vi "Main.vi"(8 "error in":errorcluster, 11 "TCP Client in":refnum<class "TCP Client.lvclass">) -> (0 "error out":errorcluster, 3 "TCP Client out":refnum<class "TCP Client.lvclass">)   [LabVIEW 2017, in "TCP Client.lvlib" / "TCP Client.lvclass"]
doc: "The <b>Queued Message Handler</b> of the Worker that owns this VI."
uses:
  TCP Client.lvclass
  C:/Program Files (x86)/National Instruments/LabVIEW 2017/vi.lib/addons/_Workers/Library/Classes/Worker/Worker.lvclass
  Initialization Data.ctl
  Response Cases.ctl
  <vilib>/addons/_Workers/Library/Case Label.ctl
  TCP Client.lvclass/TCP Client.ctl
  rql_New Connection.ctl
  <vilib>/addons/_Workers/Library/Classes/Message/Priority.ctl
  rsp_Connection Notify.ctl
  rql_Create Read Worker.ctl
  TCP Read/Initialization Data.ctl
  TCP Read/Response Cases.ctl
  <vilib>/addons/_Workers/Library/Classes/Message Queue/Message Queue.lvclass
  rwr_Connect to Server.ctl
  rqp_Send String to Server.ctl
  <vilib>/Utility/error.llb/Error Cluster From Error Code.vi
  <vilib>/ErrorRing/Error Ring.xnode
  <vilib>/addons/_Workers/Library/Classes/Worker/Worker.lvclass
  <vilib>/addons/_Workers/Library/Workers.lvlib
  <vilib>/addons/_Workers/Library/Classes/Message/Message.lvclass
  TCP Read/TCP Read.lvclass
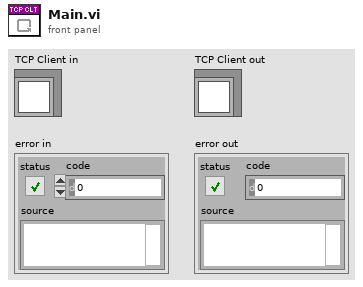
[diagram p1: front panel]
types:
  T1 = typedef "TCP Client.lvlib/TCP Client.lvclass/Initialization Data.ctl" = cluster{"Response Cases":T2}
  T2 = typedef "TCP Client.lvlib/TCP Client.lvclass/Response Cases.ctl" = cluster{"Connection Notify":T3, "Incoming Data":T3}
  T3 = typedef "Workers.lvlib/Case Label.ctl" = string
  T4 = typedef "TCP Client.lvlib/TCP Client.lvclass/rsp_Connection Notify.ctl" = cluster{"Server Name":string, "IP Address":string, "Connected?":bool}
  T5 = typedef "Workers.lvlib/Message.lvclass/Priority.ctl" = enum16{"Low", "Normal", "High"}
  T6 = typedef "TCP Client.lvlib/TCP Client.lvclass/rql_New Connection.ctl" = cluster{"Connection ID":refnum<k5>, "Server Name":string, "IP Address":string}
  T7 = typedef "TCP Client.lvlib/TCP Read.lvclass/Initialization Data.ctl" = cluster{"Response Cases":T8, "Connection ID":refnum<k5>, "Forwarding Queue":refnum<class "Message Queue.lvclass">, "Forwarding Case":T3, "Server Name":string}
  T8 = typedef "TCP Client.lvlib/TCP Read.lvclass/Response Cases.ctl" = cluster{"Connection Lost":T3}
  T9 = typedef "TCP Client.lvlib/TCP Client.lvclass/rql_Create Read Worker.ctl" = cluster{"String":string}
  T10 = typedef "TCP Client.lvlib/TCP Client.lvclass/rwr_Connect to Server.ctl" = cluster{"Client Name":string, "Server IP Address":string, "Server Port":u16}
  T11 = typedef "TCP Client.lvlib/TCP Client.lvclass/rqp_Send String to Server.ctl" = cluster{"String to Send":string}
  T12 = typedef "TCP Client.lvlib/TCP Read.lvclass/rsp_Connection Lost.ctl" = cluster{"Connection ID":refnum<k5>, "TCP Read Queue":refnum<class "Message Queue.lvclass">}
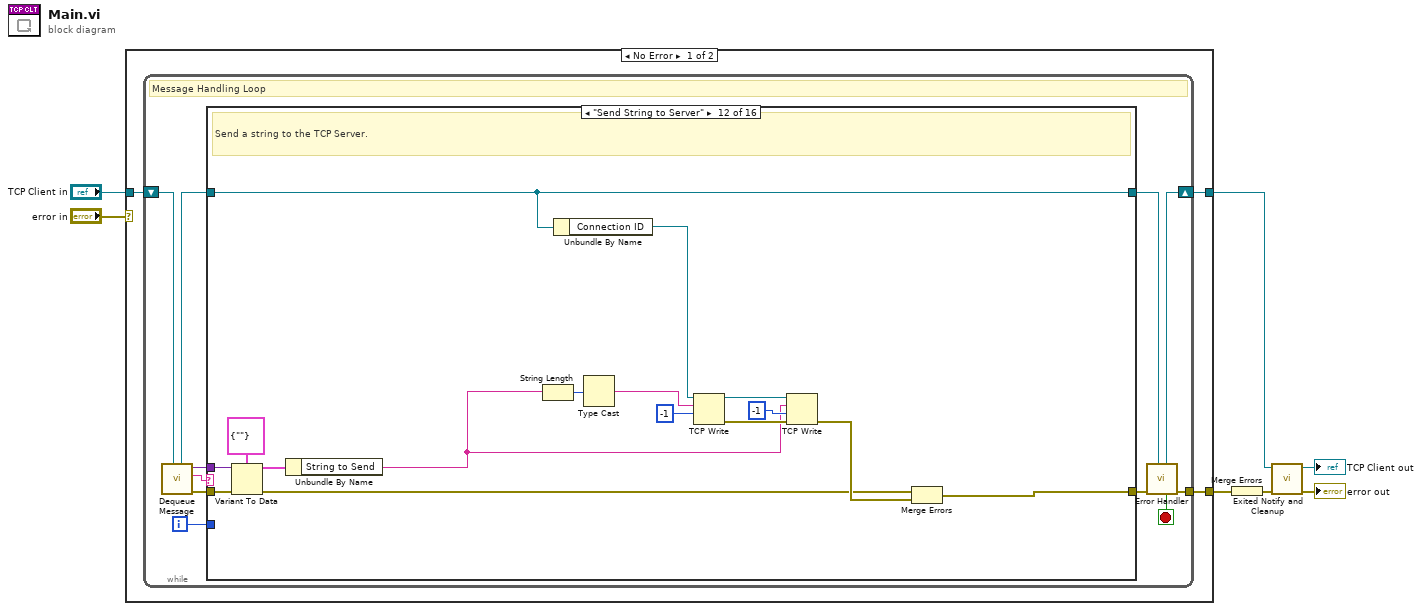
[diagram p0: block diagram]
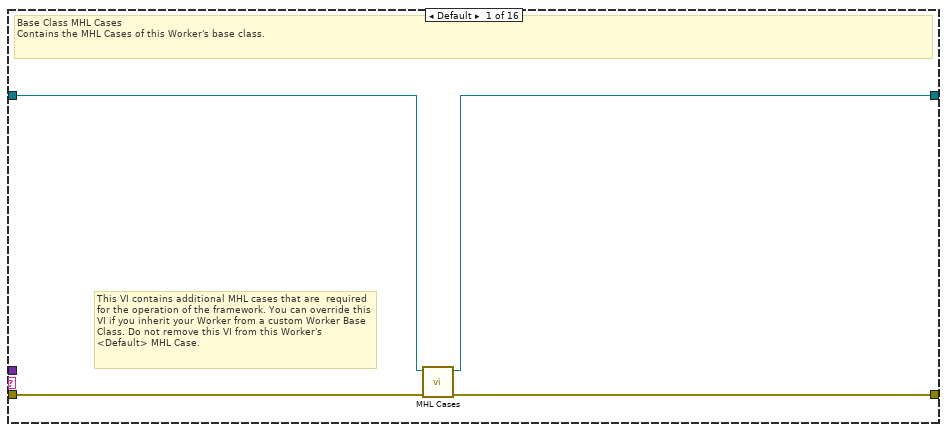
[diagram p2: hidden frame]
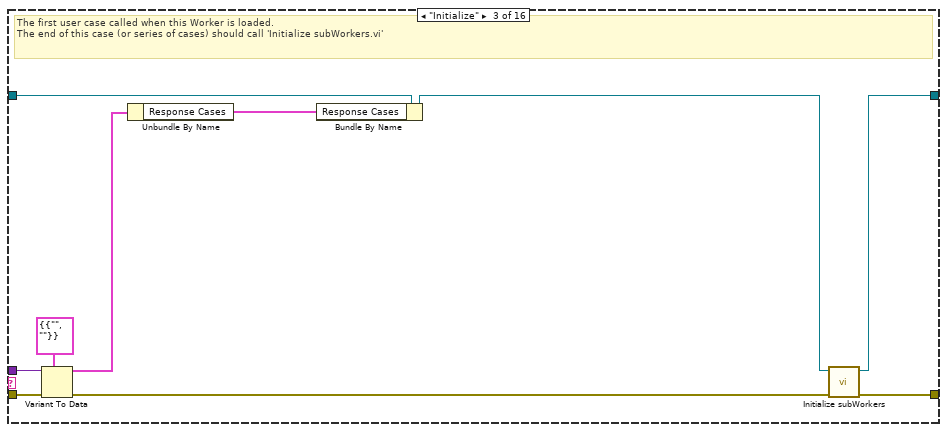
[diagram p4: hidden frame]
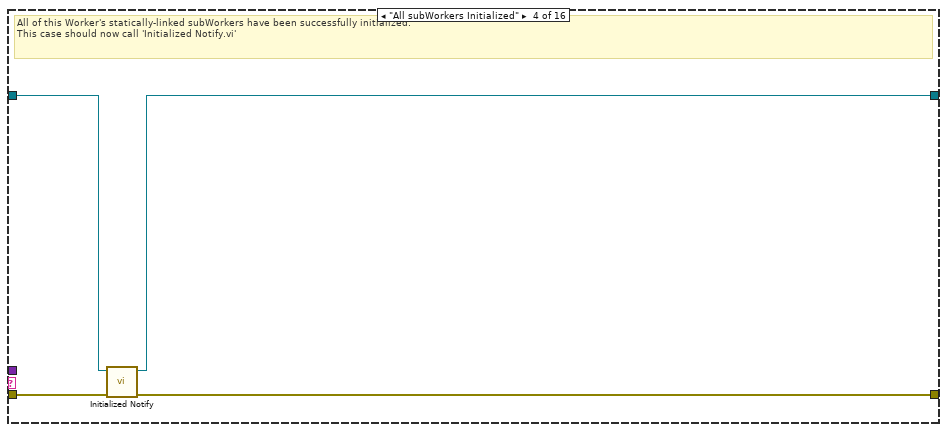
[diagram p5: hidden frame]
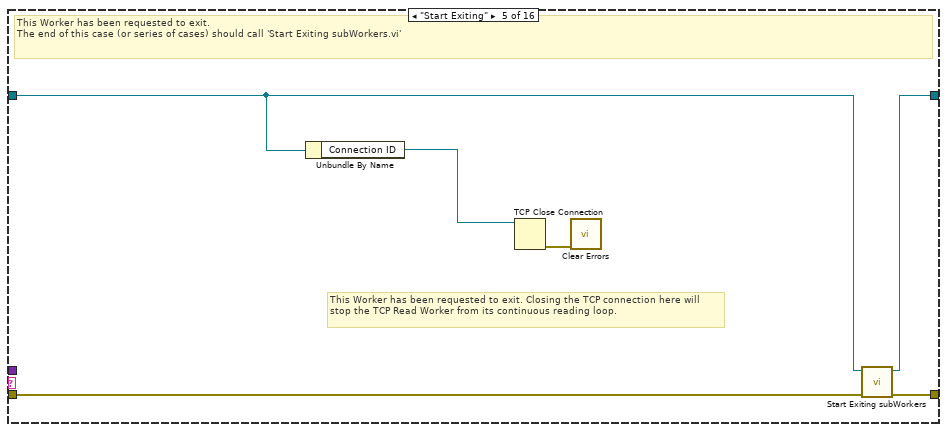
[diagram p6: hidden frame]
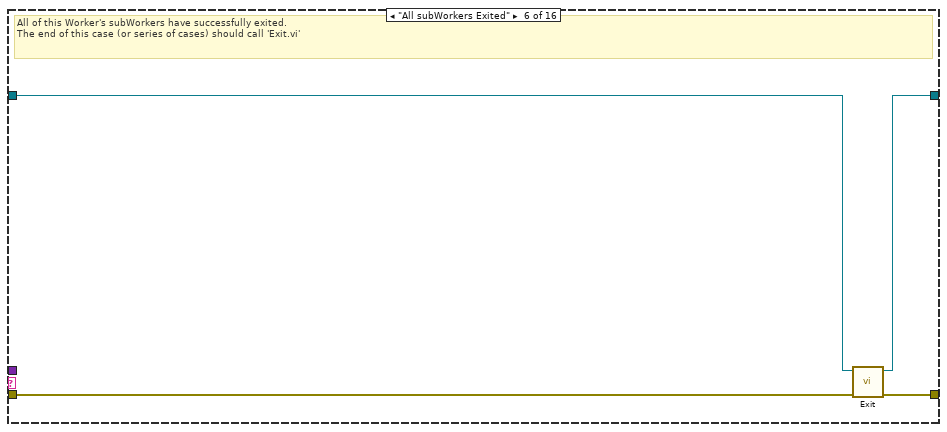
[diagram p7: hidden frame]
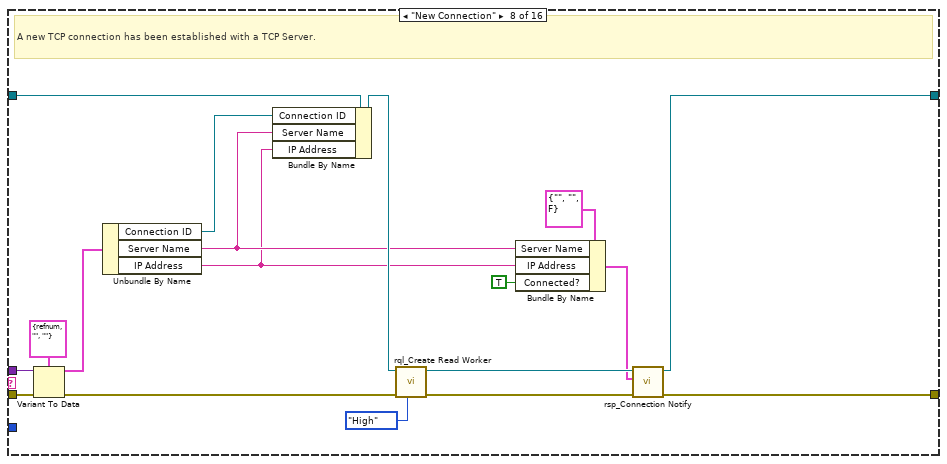
[diagram p9: hidden frame]
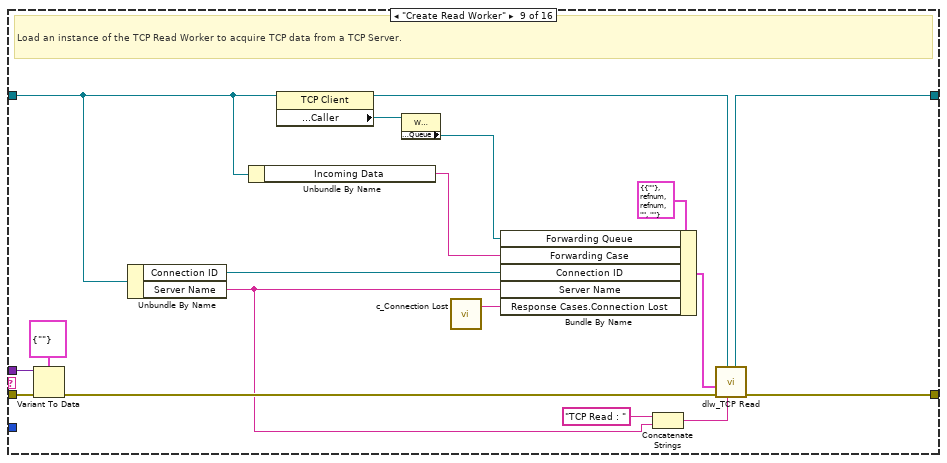
[diagram p10: hidden frame]
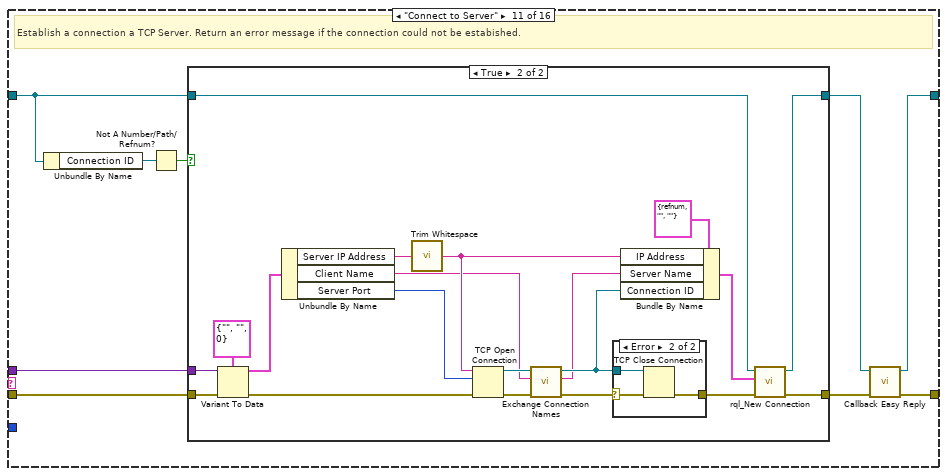
[diagram p12: hidden frame]
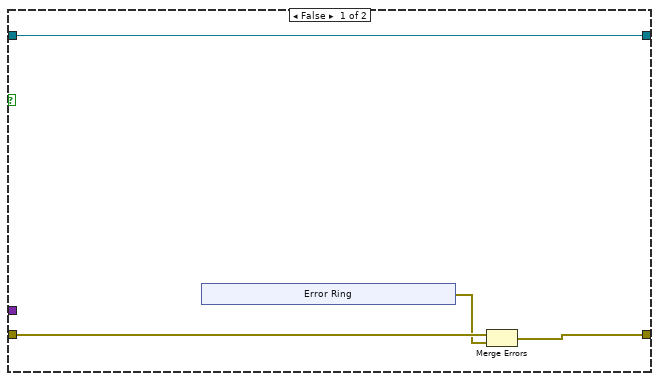
[diagram p13: hidden frame]
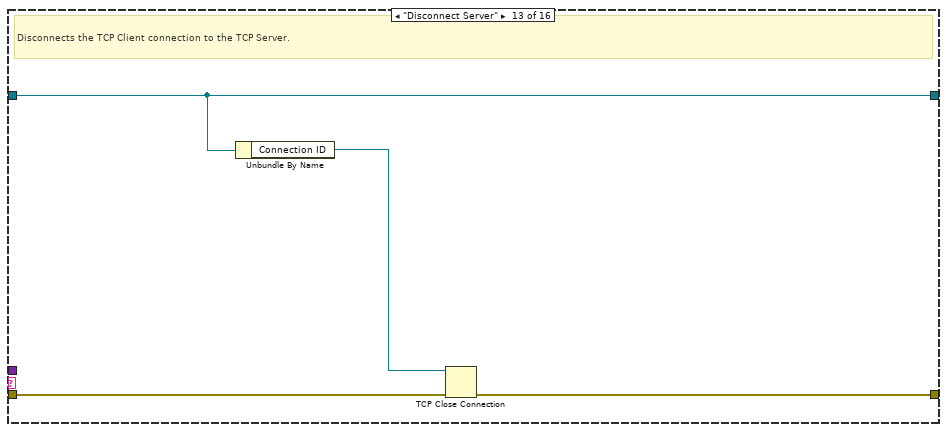
[diagram p15: hidden frame]
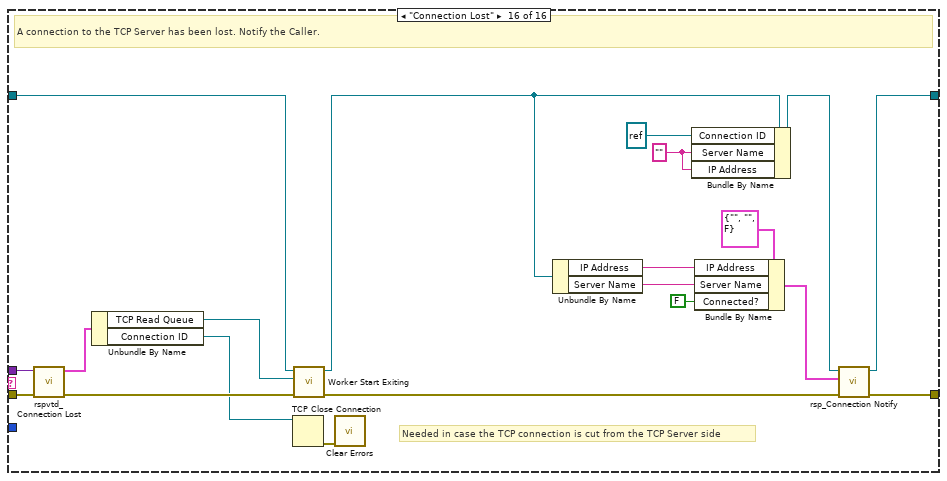
[diagram p18: hidden frame]
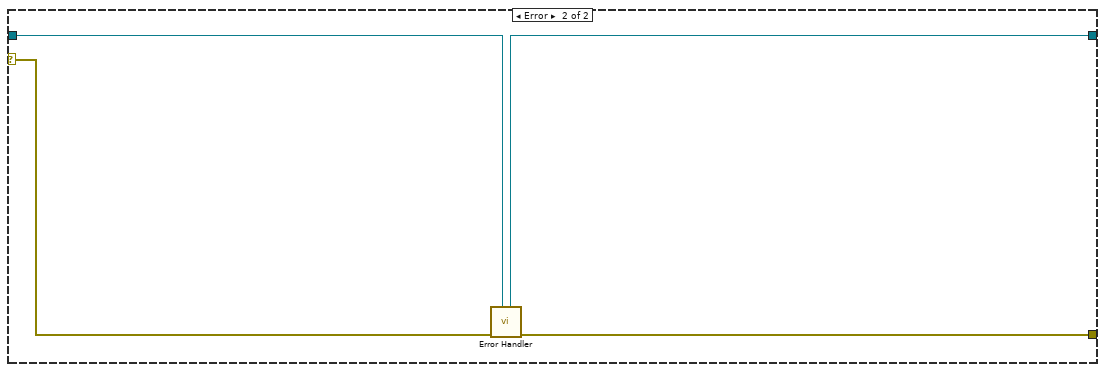
[diagram p19: hidden frame]
diagram:
  n1 = case shown="No Error" "error in" {
    tunnel: "TCP Client in" -> [w8 w178]
    tunnel: [w10 w179] -> w6
    tunnel: [w9 w177] -> w7
    selector: "error in" -> [_ w180]
    frame No Error {
      n2 = while {
        shift-right: [w19] -> w9
        shift-left: w8 -> [w21]
        tunnel: [w20] -> w10
        i -> [w12]
        stop <- w13 stop-if-true
        # "Message Handling Loop"
        n3 = call-dynamic "Dequeue Message.vi"("Worker"=w21) -> ("error out"=w18:errorcluster, "Case out"=w14:string, "Data out"=w11:variant, "Worker out"=w16:refnum<class "TCP Client.lvclass">)  [unwired: 6 in, 1 out]
        n4 = case "Worker MHL Case Structure (DO NOT CHANGE LABEL NAME)" shown="\"Send String to Server\"" w14 {
          tunnel: w18 -> [w25 w26 w35 w41 w43 w51 w53 w70 w89 w91 w100 w148 w150 w154 w155 w176]
          tunnel: [w24 w26 w37 w40 w47 w50 w53 w61 w85 w91 w97 w137 w149 w154 w155 w167] -> w17
          tunnel: w16 -> [w23 w27 w34 w39 w44 w49 w52 w71 w75 w90 w92 w145 w152 w153 w156 w171]
          tunnel: [w22 w27 w36 w38 w46 w48 w52 w59 w84 w90 w96 w145 w152 w153 w156 w170] -> w15
          tunnel: w12 -> [_ _ _ _ _ _ _ _ _ _ _ _ _ _ _ _]
          tunnel: w11 -> [_ _ w32 _ _ _ _ w67 w86 _ w98 w146 _ _ _ w175]
          frame Default {
            # "This VI contains additional MHL cases that are  required for the operation of the framework. You can override this VI if you inherit your Worker from a custom Worker Base Class. Do not remove this VI from this Worker's <Default> MHL Case."
            # "Base Class MHL Cases\nContains the MHL Cases of this Worker's base class."
            n5 = call-dynamic "MHL Cases.vi"("error in"=w25, "Worker in"=w23) -> ("error out"=w24:errorcluster, "Worker out"=w22:refnum<class "TCP Client.lvclass">)  [unwired: 8 in]
          }
          frame "------------ FRAMEWORK CASES -----------" {
            # "Start of Workers Framework Cases"
          }
          frame "Initialize" {
            # "The first user case called when this Worker is loaded.\nThe end of this case (or series of cases) should call 'Initialize subWorkers.vi'"
            n6 = Variant To Data(error in=w35, type=T1 {"Response Cases"={"Connection Notify"="", "Incoming Data"=""}} ("Cluster"), Variant=w32) -> (data=w30:T1, error out=w33:errorcluster)
            n7 = Unbundle By Name(w30) -> ("Response Cases"=w29:T2)
            n8 = Bundle By Name(cluster=w34, "Response Cases"=w29) -> (w31:refnum<class "TCP Client.lvclass">)
            n9 = call-dynamic "Initialize subWorkers.vi"("error in"=w33, "Worker"=w31) -> ("error out"=w37:errorcluster, "dup Worker out"=w36:refnum<class "TCP Client.lvclass">)  [unwired: 8 in]
          }
          frame "All subWorkers Initialized" {
            # "All of this Worker's statically-linked subWorkers have been successfully initialized.\nThis case should now call 'Initialized Notify.vi'"
            n10 = call-dynamic "Initialized Notify.vi"("error in"=w41, "Worker"=w39) -> ("error out"=w40:errorcluster, "dup Worker out"=w38:refnum<class "TCP Client.lvclass">)  [unwired: 8 in]
          }
          frame "Start Exiting" {
            # "This Worker has been requested to exit. Closing the TCP connection here will stop the TCP Read Worker from its continuous reading loop."
            # "This Worker has been requested to exit. \nThe end of this case (or series of cases) should call 'Start Exiting subWorkers.vi'"
            n11 = Unbundle By Name(w44) -> ("Connection ID"=w45:refnum<k5>)
            n12 = TCP Close Connection(connection ID=w45) -> (error out=w42:errorcluster)  [unwired: 2 in, 1 out]
            n13 = call <vilib>:"Clear Errors.vi"("error in (no error)"=w42) -> ()  [unwired: 5 in, 2 out]
            n14 = call-dynamic "Start Exiting subWorkers.vi"("error_in"=w43, "Worker"=w44) -> ("error out"=w47:errorcluster, "dup Worker out"=w46:refnum<class "TCP Client.lvclass">)  [unwired: 8 in]
          }
          frame "All subWorkers Exited" {
            # "All of this Worker's subWorkers have successfully exited. \nThe end of this case (or series of cases) should call 'Exit.vi'"
            n15 = call-dynamic "Exit.vi"("error_in"=w51, "Worker"=w49) -> ("error out"=w50:errorcluster, "dup Worker out"=w48:refnum<class "TCP Client.lvclass">)  [unwired: 8 in]
          }
          frame "------------- LOCAL API CASES -------------" {
            # "Start of Workers Local API Cases"
          }
          frame "New Connection" {
            # "A new TCP connection has been established with a TCP Server."
            n16 = Variant To Data(error in=w70, type=T6 {"Connection ID"=refnum, "Server Name"="", "IP Address"=""} ("Data"), Variant=w67) -> (data=w66:T6, error out=w69:errorcluster)
            n17 = Unbundle By Name(w66) -> ("Connection ID"=w65:refnum<k5>, "Server Name"=w56:string, "IP Address"=w54:string)
            n18 = Bundle By Name(cluster=w71, "Connection ID"=w65, "Server Name"=w56, "IP Address"=w54) -> (w63:refnum<class "TCP Client.lvclass">)
            n19 = call "rql_Create Read Worker.vi"("Message Priority"=Priority."High", "error in"=w69, "TCP Client in"=w63) -> ("error out"=w64:errorcluster, "dup TCP Client out"=w60:refnum<class "TCP Client.lvclass">)  [unwired: 7 in]
            n20 = Bundle By Name(cluster=T4 {"Server Name"="", "IP Address"="", "Connected?"=FALSE} ("Data in"), "Server Name"=w56, "IP Address"=w54, "Connected?"=TRUE) -> (w57:T4)
            n21 = call "rsp_Connection Notify.vi"("error in"=w64, "Data in"=w57, "TCP Client in"=w60) -> ("error out"=w61:errorcluster, "dup TCP Client out"=w59:refnum<class "TCP Client.lvclass">)  [unwired: 7 in]
          }
          frame "Create Read Worker" {
            # "Load an instance of the TCP Read Worker to acquire TCP data from a TCP Server."
            n22 = Variant To Data(error in=w89, type=T9 {"String"=""} ("Data"), Variant=w86) -> (error out=w88:errorcluster)  [unwired: 1 out]
            n23 = Unbundle By Name(w75) -> ("Connection ID"=w77:refnum<k5>, "Server Name"=w76:string)
            n24 = Unbundle By Name(w75) -> ("Incoming Data"=w74:T3)
            n25 = property class="TCP Client"(reference=w75) -> (reference out=w79:refnum<class "TCP Client.lvclass">, "Accessors:Read:Public API:Caller"=w78:refnum<class "Worker.lvclass">)  [unwired: 1 in, 1 out]
            n26 = property class="Worker.lvclass"(reference=w78) -> ("Accessors:Read:Public API:Queue"=w72:refnum<class "Message Queue.lvclass">)  [unwired: 1 in, 2 out]
            n27 = call "c_Connection Lost.vi"() -> ("Case Label"=w73:T3)  [unwired: 1 in]
            n28 = Bundle By Name(cluster=T7 {"Response Cases"={"Connection Lost"=""}, "Connection ID"=refnum, "Forwarding Queue"=refnum, "Forwarding Case"="", "Server Name"=""} ("Initialization Data"), "Forwarding Queue"=w72, "Forwarding Case"=w74, "Connection ID"=w77, "Server Name"=w76, "Response Cases.Connection Lost"=w73) -> (w82:T7)
            n29 = Concatenate Strings("TCP Read : " ("Worker Alias"), w76) -> (w80:string)
            n30 = call "dlw_TCP Read.vi"("Worker Alias"=w80, "Caller in"=w79, "error in"=w88, "Initialization Data"=w82) -> ("error out"=w85:errorcluster, "dup Caller out"=w84:refnum<class "TCP Client.lvclass">)  [unwired: 5 in, 1 out]
          }
          frame "------------- PUBLIC API CASES -------------" {
            # "Start of Workers Public API Cases"
          }
          frame "Connect to Server" {
            # "Establish a connection a TCP Server. Return an error message if the connection could not be estabished."
            n31 = Unbundle By Name(w92) -> ("Connection ID"=w94:refnum<k5>)
            n32 = Not A Number/Path/Refnum?(number/path/refnum=w94) -> (NaN/Path/Refnum?=w93:bool)
            n33 = case shown="True" w93 {
              tunnel: w100 -> [w103 w128]
              tunnel: [w102 w118] -> w99
              tunnel: w98 -> [_ w126]
              tunnel: [w104 w116] -> w95
              tunnel: w92 -> [w104 w117]
              frame False {
                n34 = xnode "Error Ring"() -> ("error out"=w101:errorcluster)
                n35 = Merge Errors(w103, w101) -> (w102:errorcluster)
              }
              frame True {
                n36 = Variant To Data(error in=w128, type=T10 {"Client Name"="", "Server IP Address"="", "Server Port"=0} ("Data"), Variant=w126) -> (data=w125:T10, error out=w122:errorcluster)
                n37 = Unbundle By Name(w125) -> ("Server IP Address"=w123:string, "Client Name"=w110:string, "Server Port"=w124:u16)
                n38 = call <vilib>:"Trim Whitespace.vi"("string"=w123) -> ("trimmed string"=w113:string)  [unwired: 1 in]
                n39 = TCP Open Connection(address=w113, remote port or service name=w124) -> (connection ID=w121:refnum<k5>)  [unwired: 2 in, 2 out]
                n40 = call "Exchange Connection Names.vi"("error in (no error)"=w122, "Client Name in"=w110, "connection ID"=w121) -> ("error out"=w120:errorcluster, "Server Name out"=w111:string, "connection out"=w112:refnum<k5>)  [unwired: 6 in]
                n41 = case shown="Error" w120 {
                  selector: w120 -> [w129 w130]
                  tunnel: [w129 w132] -> w119
                  tunnel: w112 -> [_ w131]
                  frame No Error {
                  }
                  frame Error {
                    n42 = TCP Close Connection(connection ID=w131, error in (no error)=w130) -> (error out=w132:errorcluster)  [unwired: 1 in, 1 out]
                  }
                }
                n43 = Bundle By Name(cluster=T6 {"Connection ID"=refnum, "Server Name"="", "IP Address"=""} ("Data in"), "IP Address"=w113, "Server Name"=w111, "Connection ID"=w112) -> (w114:T6)
                n44 = call "rql_New Connection.vi"("error in"=w119, "Data in"=w114, "TCP Client in"=w117) -> ("error out"=w118:errorcluster, "dup TCP Client out"=w116:refnum<class "TCP Client.lvclass">)  [unwired: 7 in]
              }
            }
            n45 = call-dynamic "Callback Easy Reply.vi"("error in"=w99, "Worker"=w95) -> ("error out"=w97:errorcluster, "dup Worker out"=w96:refnum<class "TCP Client.lvclass">)  [unwired: 8 in]
          }
          frame "Send String to Server" {
            # "Send a string to the TCP Server."
            n46 = Variant To Data(error in=w148, type=T11 {"String to Send"=""} ("Data"), Variant=w146) -> (data=w135:T11, error out=w133:errorcluster)
            n47 = Unbundle By Name(w135) -> ("String to Send"=w134:string)
            n48 = String Length(string=w134) -> (length=w139:i32)
            n49 = Unbundle By Name(w145) -> ("Connection ID"=w140:refnum<k5>)
            n50 = Type Cast(x=w139) -> (*(type *) &x=w138:string)  [unwired: 1 in]
            n51 = TCP Write(connection ID=w140, data in=w138, 9:-1 ("timeout ms (25000)")) -> (connection ID out=w143:refnum<k5>, error out=w144:errorcluster)  [unwired: 1 in, 1 out]
            n52 = TCP Write(connection ID=w143, data in=w134, error in (no error)=w144, 9:-1 ("timeout ms (25000)")) -> (error out=w136:errorcluster)  [unwired: 2 out]
            n53 = Merge Errors(w133, w136) -> (w137:errorcluster)
          }
          frame "Disconnect Server" {
            # "Disconnects the TCP Client connection to the TCP Server."
            n54 = Unbundle By Name(w152) -> ("Connection ID"=w151:refnum<k5>)
            n55 = TCP Close Connection(connection ID=w151, error in (no error)=w150) -> (error out=w149:errorcluster)  [unwired: 1 in, 1 out]
          }
          frame "------------- RESPONSE CASES --------------" {
            # "Start of Workers Response Cases"
          }
          frame "~~~~~~~~~~ TCP Read ~~~~~~~~~~~~ " {
          }
          frame "Connection Lost" {
            w159 = "" ("Server Name")
            # "Needed in case the TCP connection is cut from the TCP Server side"
            # "A connection to the TCP Server has been lost. Notify the Caller."
            n56 = call "rspvtd_Connection Lost.vi"("error in"=w176, "Data in"=w175) -> ("error out"=w168:errorcluster, "Data out"=w169:T12)  [unwired: 8 in]
            n57 = Unbundle By Name(w169) -> ("TCP Read Queue"=w173:refnum<class "Message Queue.lvclass">, "Connection ID"=w157:refnum<k5>)
            n58 = TCP Close Connection(connection ID=w157) -> (error out=w172:errorcluster)  [unwired: 2 in, 1 out]
            n59 = call-dynamic "Worker Start Exiting.vi"("error_in"=w168, "Message Queue"=w173, "Worker"=w171) -> ("error out"=w174:errorcluster, "dup Worker out"=w161:refnum<class "TCP Client.lvclass">)  [unwired: 7 in]
            n60 = call <vilib>:"Clear Errors.vi"("error in (no error)"=w172) -> ()  [unwired: 5 in, 2 out]
            n61 = Unbundle By Name(w161) -> ("IP Address"=w158:string, "Server Name"=w160:string)
            n62 = Bundle By Name(cluster=w161, "Connection ID"=refnum<k5> refnum, "Server Name"=w159, "IP Address"=w159) -> (w166:refnum<class "TCP Client.lvclass">)
            n63 = Bundle By Name(cluster=T4 {"Server Name"="", "IP Address"="", "Connected?"=FALSE} ("Data in"), "IP Address"=w158, "Server Name"=w160, "Connected?"=FALSE) -> (w164:T4)
            n64 = call "rsp_Connection Notify.vi"("error in"=w174, "Data in"=w164, "TCP Client in"=w166) -> ("error out"=w167:errorcluster, "dup TCP Client out"=w170:refnum<class "TCP Client.lvclass">)  [unwired: 7 in]
          }
        }
        n65 = call-dynamic "Error Handler.vi"("Worker"=w15, "error_in"=w17) -> ("error out"=w20:errorcluster, "Stop Loop"=w13:bool, "Worker out"=w19:refnum<class "TCP Client.lvclass">)  [unwired: 7 in]
      }
    }
    frame Error {
      n66 = call-dynamic "Error Handler.vi"("Worker"=w178, "error_in"=w180) -> ("error out"=w179:errorcluster, "Worker out"=w177:refnum<class "TCP Client.lvclass">)  [unwired: 7 in, 1 out]
    }
  }
  n67 = Merge Errors(w6) -> (w3:errorcluster)
  n68 = call-dynamic "Exited Notify and Cleanup.vi"("error_in"=w3, "Worker"=w7) -> ("error out"=→"error out":errorcluster, "dup Worker out"=→"TCP Client out":refnum<class "TCP Client.lvclass">)  [unwired: 8 in]
